vi "Main-Strech DNA-OneDirectionOnly_ver2_YCC.vi"(4 "Avg points":i32=120, 5 "Save Data?":bool, 6 "Who's Data":enum16{"YCC", "PYW", "LCH", "YYH"}(ring), 7 "Set LaserPower (mV)":dbl=-4500.0 format="%0.2f", 8 "File name add to the end \n(laser power-height)":string="FA-h300-1-1", 9 "Record scan rate  (um/s)":dbl=3.0 format="%.3f", 10 "range  (um)":dbl=2.9499999999999975 format="%.3f", 11 "T=X\nF=Y":bool=TRUE) -> (3 "Stage-QPD Graph":T4(graph))   [LabVIEW 2014]
uses:
  Main-Calibration/WLC fitting/SubVI/WLC-Fitting Cluster.ctl
  <vilib>/Analysis/baseanly.llb/Mean (DBL).vi
  <vilib>/Analysis/NI_AALBase.lvlib
panel:
  out "center":dbl
  out "avg. Step (nm)":dbl
  in  "WLC fitting?":bool
  in  "Force offset":dbl=800.0
  in  "Length offset":dbl=700.0
  in  "Filter type":T1(ring)=enum."F+S-window avg"
  in  "trap height(nm)":dbl=300.0
  out "Laser Lock?":bool
  in  "xDNA cut outside":dbl=3000.0
  in  "Fitting Cluster 2":T2={"cr (um)"=0.0, "yr (V)"=0.0, "trap height(nm)"=0.0, "bead radius(nm)"=520.0, "Length offset"=0.0, "Upper Force(pN)"=0.0, "cr shift (nm)"=0.0, "yr shift (mV)"=0.0, "LaserPower (mW)"=0.0, "conversion factor (V/um)"=0.0, "Stiffness (pN/nm)"=0.0154, "xDNA cut outside"=0.0, "Lower Force(pN)"=5.0, "c for zbd"=0.0}
  out "True rate?":bool
  in  "no fec":bool=TRUE
  in  "Avg. time delay (ms)":dbl=18.0
  in  "Use avg delay?":bool=TRUE
  out "delay time between F and U (ms)":dbl
  in  "no Record scan rate  (um/s)":dbl=2.0
  out "Fold QPD Signal (V) 2":dbl[](array[numeric])
  out "Fold Stage Position (um) 2":dbl[](array[numeric])
  out "Folded-Force":dbl[](array[numeric])
  out "Folded-xDNA":dbl[](array[numeric])
  out "Unfolded-Force":dbl[](array[numeric])
  out "Unfolded-xDNA":dbl[](array[numeric])
  out "Filtered QPD Array":dbl[][](array[numeric])
  out "Filtered Stage Array":dbl[][](array[numeric])
  out "Save to File Name Indicator":string
  out "Save to Path Indicator":path
  out "initial position offset after move":dbl[](array[numeric])
  out "Avg. to Hz":dbl
  out "Fold QPD Signal (V)":dbl[](array[numeric])
  out "Unfold QPD Signal (V)":dbl[](array[numeric])
  out "Fold Stage Position (um)":dbl[](array[numeric])
  out "Unfold Stage Position (um)":dbl[](array[numeric])
  in  "Tab Control":T3(tab)
  out "Stage-QPD Graph 3":T4(graph)
  out "Stage-QPD Graph 2":T4(graph)
  out "Unfolded Graph":cluster{dbl[], dbl[]}(graph)
  out "Folded Graph":cluster{dbl[], dbl[]}(graph)
  out "Unfolded+Folded Graph":T5(graph)
  out "Unfolded Fitting Graph":T6(graph)
  in  "initial parameters for eWLC (Lp,Lc,K)":dbl[](array[numeric])=[45.0, 1800.0, 1200.0]
  in  "initial parameters for marko (Lp,Lc)":dbl[](array[numeric])=[40.0, 1800.0]
  out "best fit parameters\n(Lp,Lc)":dbl[](array[numeric])
  out "best fit parameters\n(Lp,Lc,K)":dbl[](array[numeric])
  out "r^2":dbl
  out "r^2  2":dbl
  in  "eWLC?":bool
  out "Trace direction":bool[](array[boolean])=[FALSE, TRUE, TRUE, FALSE]
  out "Real initial position (um)":dbl format="%0.5f"
  in  "Toward first ?\nT=+, F=-":bool
  in  "Record Mode \npath(1,2)":bool[](array[boolean])=[TRUE, TRUE, FALSE, FALSE]
  in  "Sampling rate":dbl=32000.0 format="%0.2f"
  # "3.8 for full range"
  # "range=3.1um & 4 um/s\n-2000 m¢ä for activead"
  # "avg delay= 33ms\n20181223 ·s¬°18ms"
  # "3281-h300-sp40-RecA-ATPrS-6"
  # "3281-h300-m51 BRC4 2uM-Ca-ATP-1-8"
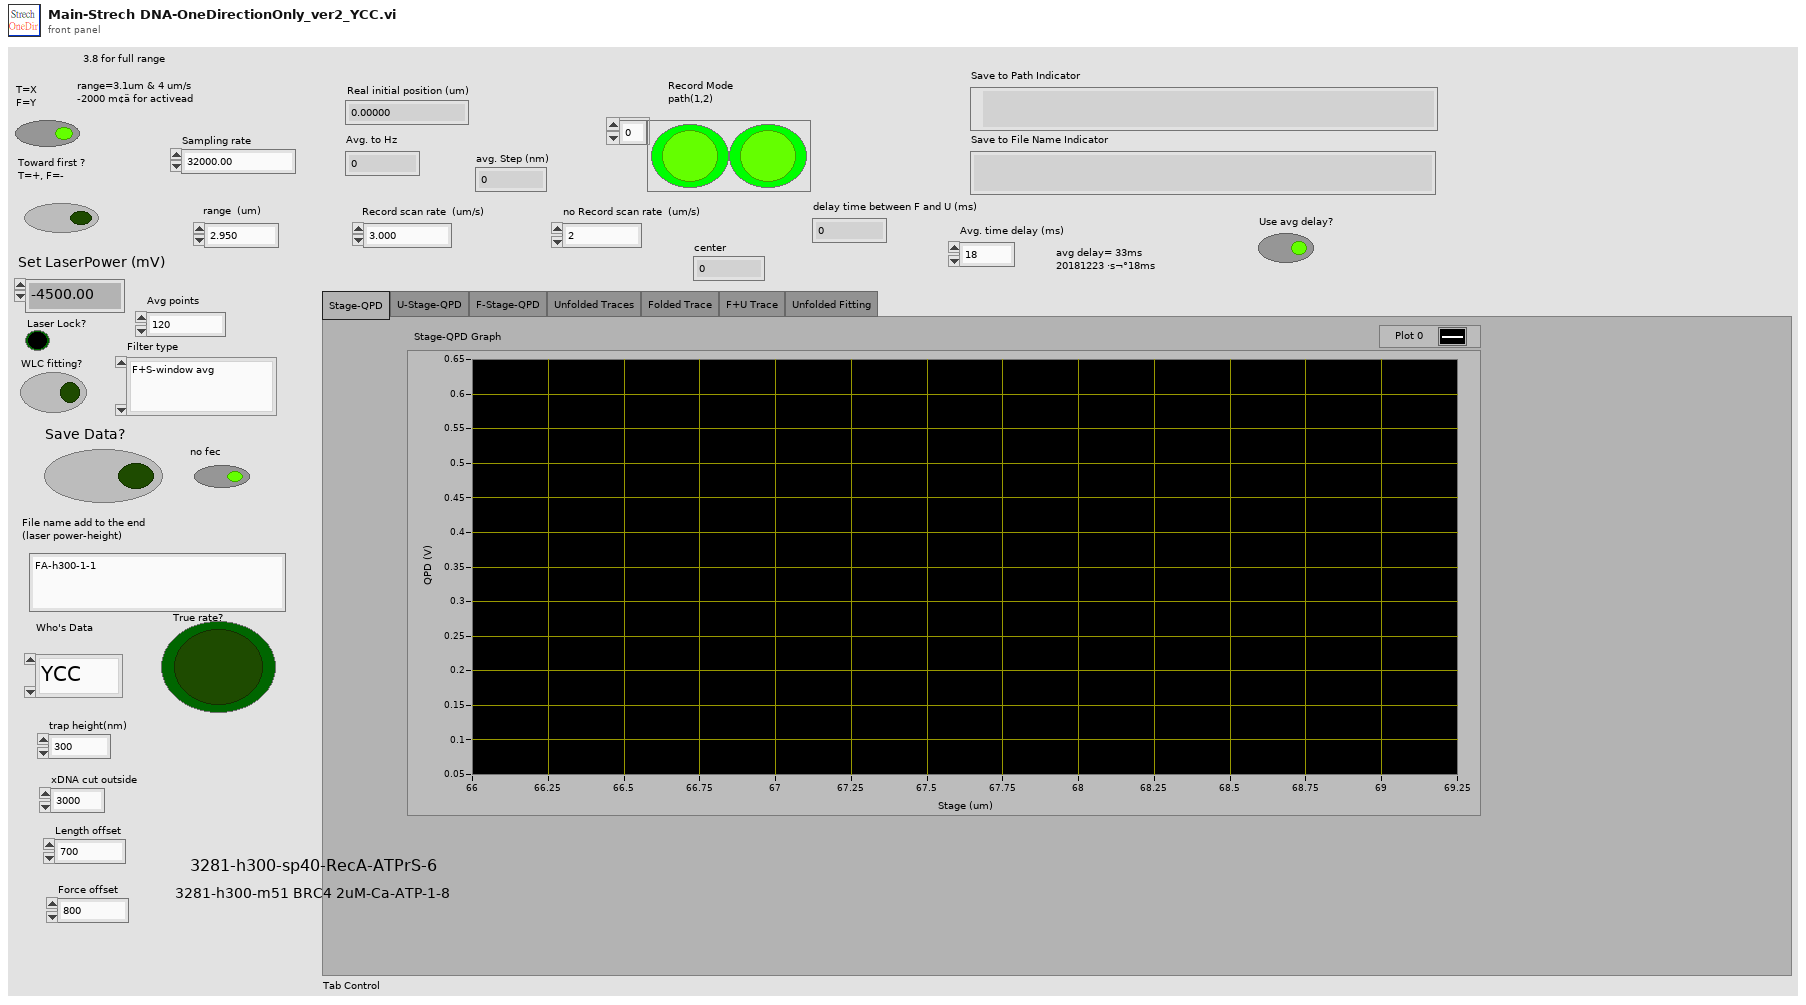
[diagram p1: front panel]
types:
  T1 = enum16{"Fixed-window avg", "Moving-window avg", "F+S-window avg", "S-G filter", "Fixed-window Median", "Moving-window Median "}
  T2 = typedef "WLC-Fitting Cluster.ctl" = cluster{"cr (um)":dbl, "yr (V)":dbl, "trap height(nm)":dbl, "bead radius(nm)":dbl, "Length offset":dbl, "Upper Force(pN)":dbl, "cr shift (nm)":dbl, "yr shift (mV)":dbl, "LaserPower (mW)":dbl, "conversion factor (V/um)":dbl, "Stiffness (pN/nm)":dbl, "xDNA cut outside":dbl, "Lower Force(pN)":dbl, "c for zbd":dbl}
  T3 = enum32{"Stage-QPD", "U-Stage-QPD", "F-Stage-QPD", "Unfolded Traces", "Folded Trace", "F+U Trace", "Unfolded Fitting"}
  T4 = cluster{"Fold Stage Position (um)":dbl[], "Fold QPD Signal (V)":dbl[]}
  T5 = cluster{"Filtered Stage Array":dbl[], "Filtered QPD Array":dbl[]}[]
  T6 = cluster{"best nonlinear fit for Extension (nm)":dbl[], "Force to fit":dbl[]}[]
  T7 = enum16{"Custom", "Centering", "1000 mV", "4500 mV"}
  T8 = cluster{"best nonlinear fit for Extension (nm)":dbl[], "Force to fit":dbl[]}
  T9 = cluster{"Unfolded-xDNA":dbl[], "Unfolded-Force":dbl[]}
  T10 = cluster{"Extension to fit":dbl[], "best nonlinear fit for Force (pN)":dbl[]}
  T11 = cluster{"Folded-xDNA":dbl[], "Folded-Force":dbl[]}
  T12 = cluster{"Folded-xDNA":dbl[], "Folded-Force":dbl[]}[]
  T13 = cluster{"Unfold Stage Position (um)":dbl[], "Unfold QPD Signal (V)":dbl[]}
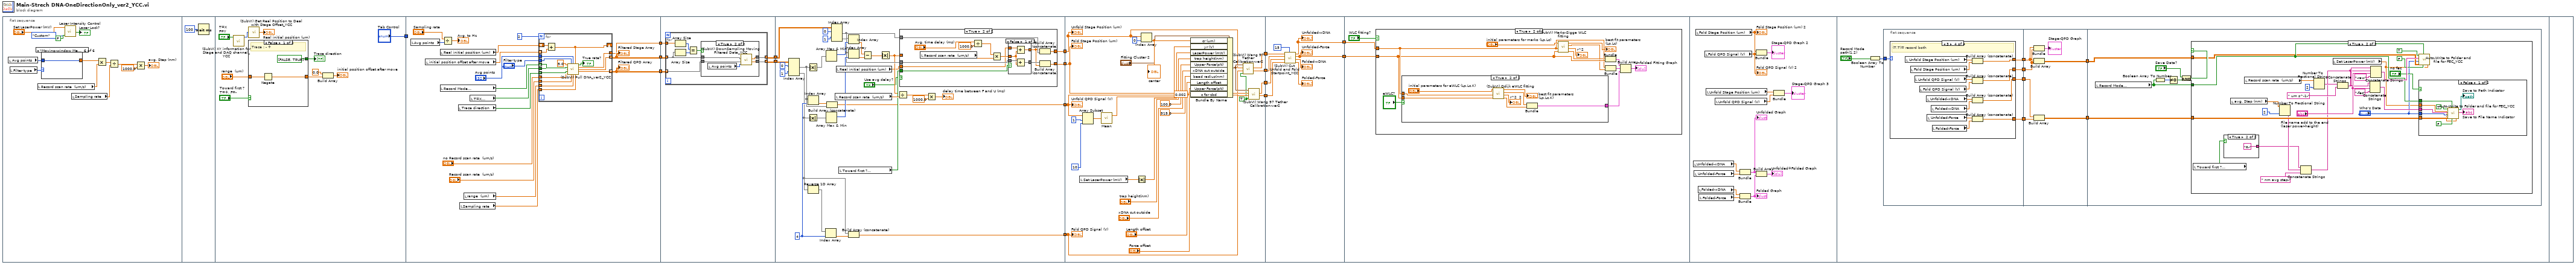
[diagram p0: block diagram]
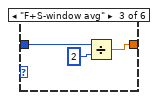
[diagram p4: hidden frame]
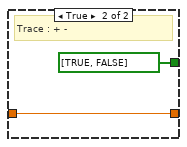
[diagram p7: hidden frame]
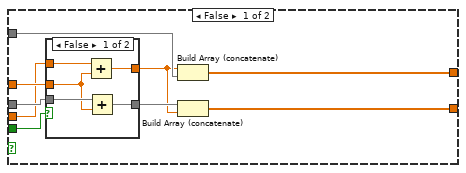
[diagram p9: hidden frame]
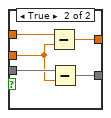
[diagram p10: hidden frame]
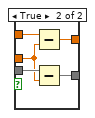
[diagram p11: hidden frame]
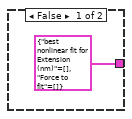
[diagram p13: hidden frame]
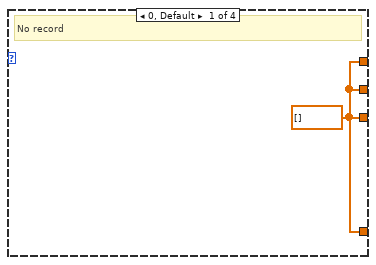
[diagram p14: hidden frame]
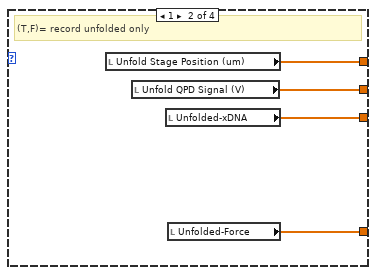
[diagram p15: hidden frame]
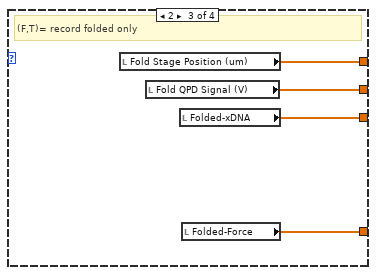
[diagram p16: hidden frame]
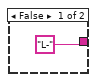
[diagram p18: hidden frame]
diagram:
  n1 = flat-sequence {
    tunnel: ["Tab Control"] -> w16
    tunnel: [w62] -> w5
    tunnel: [w61] -> w7
    tunnel: w16 -> [_]
    tunnel: [w54] -> w3
    tunnel: w7 -> [w92]
    tunnel: [w89] -> w6
    tunnel: w5 -> [w93]
    tunnel: [w90] -> w4
    tunnel: w3 -> [w91]
    tunnel: w6 -> [w136]
    tunnel: w4 -> [w139]
    tunnel: [w121] -> w11
    tunnel: [w116] -> w10
    tunnel: [w115] -> w9
    tunnel: [w118] -> w8
    tunnel: [w207] -> w15
    tunnel: [w206] -> w14
    tunnel: [w205] -> w13
    tunnel: [w204] -> w12
    tunnel: w11 -> [w203]
    tunnel: w10 -> [w192]
    tunnel: w9 -> [w202]
    tunnel: w8 -> [w193]
    tunnel: w15 -> [w218]
    tunnel: w14 -> [w217]
    tunnel: w13 -> [w216]
    tunnel: w12 -> [w214]
    tunnel: [w211] -> w2
    tunnel: [w210] -> w1
    tunnel: w2 -> [w221]
    tunnel: w1 -> [w220]
    frame #0 {
      n2 = local read "Avg points"() -> (w18:i32)
      n3 = local read "Filter type"() -> (w20:T1)
      n4 = local read "Record scan rate  (um/s)"() -> (w26:dbl)
      n5 = case shown="\"Moving-window Median \"" w20 {
        tunnel: [w30 w31 w32 w35 w36 w37] -> w19
        tunnel: w18 -> [w30 w31 w34 w35 w36 w37]
        frame "Fixed-window avg", Default {
        }
        frame "Moving-window avg" {
        }
        frame "F+S-window avg" {
          n6 = Divide(x=w34, y=2) -> (x/y=w32:dbl)
        }
        frame "S-G filter" {
        }
        frame "Fixed-window Median" {
        }
        frame "Moving-window Median " {
        }
      }
      n7 = call "Laser Intensity Control.vi"("Close?"=FALSE, "Enum"=T7."Custom", "Intensity Control, 0~-7000 (mV)"="Set LaserPower (mV)") -> ("Laser Lock?"=→"Laser Lock?":bool)  [unwired: 4 in]
      n8 = local read "Sampling rate"() -> (w24:dbl)
      n9 = Multiply(x=w19, y=w26) -> (x*y=w25:dbl)
      n10 = Divide(x=w25, y=w24) -> (x/y=w23:dbl)
      n11 = Multiply(x=w23, y=1000.0) -> (x*y=→"avg. Step (nm)":dbl)
    }
    frame #1 {
      n12 = Wait (ms)(milliseconds to wait=u32 100) -> ()  [unwired: 1 out]
    }
    frame #2 {
      n13 = call "(SubVI) XY information for Stage and DAQ channel_YCC.vi"("T=X\nF=Y"="T=X\nF=Y") -> ("Axis"=w46:i32)  [unwired: 3 in, 1 out]
      n14 = call "(SubVI) Get Real Position to Deal with Stage Offset_YCC.vi"("Axis"=w46) -> ("Real Current Commanded position (um)"=→"Real initial position (um)":dbl)  [unwired: 3 in, 1 out]
      n15 = case shown="False" "Toward first ?\nT=+, F=-" {
        tunnel: [bool[] [FALSE, TRUE] bool[] [TRUE, FALSE]] -> w44
        tunnel: "range  (um)" -> [w50 w52]
        tunnel: [w49 w52] -> w39
        frame False {
          # "Trace : - +"
          n16 = Negate(x=w50) -> (-x=w49:dbl)
        }
        frame True {
          # "Trace : + -"
        }
      }
      "Trace direction" <- w44
      n17 = Build Array(0.0, w39) -> (→"initial position offset after move":dbl[])
    }
    frame #3 {
      n18 = local read "Avg points"() -> (w66:i32)
      n19 = local read "initial position offset after move"() -> (w63:dbl[])
      n20 = local read "Real initial position (um)"() -> (w57:dbl)
      n21 = local read "Record Mode \npath(1,2)"() -> (w68:bool[])
      n22 = Divide(x="Sampling rate", y=w66) -> (x/y=→"Avg. to Hz":dbl)
      n23 = local read "Trace direction"() -> (w69:bool[])
      n24 = local read "Sampling rate"() -> (w58:dbl)
      n25 = local read "range  (um)"() -> (w64:dbl)
      n26 = local read "T=X\nF=Y"() -> (w70:bool)
      n27 = for {
        N: 2 -> [_]
        tunnel: "Avg points" -> [w88]
        tunnel: w68 -> [w87] mode=indexing
        tunnel: w70 -> [w86]
        tunnel: w69 -> [w79] mode=indexing
        tunnel: w58 -> [w85]
        tunnel: "Record scan rate  (um/s)" -> [w84]
        tunnel: w64 -> [w83]
        tunnel: [w73] -> w62 mode=indexing
        tunnel: [w74] -> w61 mode=indexing
        shift-right: [w80] -> _
        shift-left: w57 -> [w81]
        tunnel: w63 -> [w82] mode=indexing
        tunnel: "no Record scan rate  (um/s)" -> [w78]
        tunnel: "Filter type" -> [w75]
        tunnel: [w72] -> w54
        n28 = Add(x=w81, y=w82) -> (x+y=w80:dbl)
        n29 = call "(SubVI) Pull DNA_ver2_YCC.vi"("waiting time per point (ms)\nrange from 5ms to 0.167 ms"=5.0 ("waiting time per point (ms)\nrange from 5ms to 0.167 ms"), "Filter type"=w75, "Avg points"=w88, "Real initial position (um)"=w80, "Record?"=w87, "T=X\nF=Y"=w86, "Toward  ?\nT=+, F=-"=w79, "no Record scan rate  (um/s)"=w78, "Record scan rate  (um/s)"=w84, "range  (um)"=w83, "Sampling rate"=w85) -> ("True rate?"=→"True rate?":bool, "Raw Stage Array"=w72:dbl[], "Filtered Stage Array"=w73:dbl[], "Filtered QPD Array"=w74:dbl[])  [unwired: 1 in]
      }
      "Filtered Stage Array" <- w62
      "Filtered QPD Array" <- w61
    }
    frame #4 {
      n30 = for {
        tunnel: w93 -> [w96] mode=indexing
        tunnel: w92 -> [w98] mode=indexing
        tunnel: w91 -> [w97]
        tunnel: [w95] -> w90 mode=indexing
        tunnel: [w94] -> w89 mode=indexing
        n31 = Array Size(array=w97) -> (size(s)=w99:i32)
        n32 = Array Size(array=w96) -> (size(s)=w100:i32)
        n33 = Equal?(x=w99, y=w100) -> (x = y?=w101:bool)
        n34 = case shown="True" w101 {
          tunnel: w96 -> [w103 w107]
          tunnel: w98 -> [w102 w106]
          tunnel: [w102 w105] -> w94
          tunnel: [w103 w104] -> w95
          frame False {
          }
          frame True {
            n35 = local read "Avg points"() -> (w108:i32)
            n36 = call "(SubVI) DownSampling Moving Filtered Data_YCC.vi"("data# reduce factor"=w108, "Moving Filtered QPD data"=w106, "Moving Filtered Stage data"=w107) -> ("DownSampling QPD"=w105:dbl[], "DownSampling Stage"=w104:dbl[])  [unwired: 3 in]
          }
        }
      }
    }
    frame #5 {
      w113 = 4 ("index")
      n37 = Index Array(array=w136, index (row) #1=0 ("index (row)"), index (row) #2=1 ("index (row)")) -> (element #1=w114:dbl[], element #2=w110:dbl[])  [unwired: 2 in]
      n38 = Absolute Value(x=w114) -> (abs(x)=w135:dbl[])
      n39 = Absolute Value(x=w110) -> (abs(x)=w134:dbl[])
      n40 = Index Array(array=w114, index=w113) -> (element=w112:dbl)
      n41 = Reverse 1D Array(array=w110) -> (reversed array=w109:dbl[])
      n42 = Index Array(array=w109, index=w113) -> (element=w111:dbl)
      n43 = Array Max & Min(array=w135) -> (max index (indices)=w131:i32)  [unwired: 3 out]
      n44 = Array Max & Min(array=w134) -> (max index (indices)=w130:i32)  [unwired: 3 out]
      n45 = Build Array (concatenate)(w112, w114) -> (w116:dbl[])
      n46 = Index Array(array=w139, index (row) #1=0 ("index (row)"), index (row) #2=1 ("index (row)")) -> (element #1=w119:dbl[], element #2=w123:dbl[])  [unwired: 2 in]
      n47 = local read "Record scan rate  (um/s)"() -> (w125:dbl)
      n48 = local read "Real initial position (um)"() -> (w117:dbl)
      n49 = local read "Toward first ?\nT=+, F=-"() -> (w124:bool)
      n50 = Index Array(array=w119, index=w131) -> (element=w133:dbl)
      n51 = Index Array(array=w123, index=w130) -> (element=w132:dbl)
      n52 = Build Array (concatenate)(w110, w111) -> (w115:dbl[])
      n53 = Subtract(x=w133, y=w132) -> (x-y=w126:dbl)
      n54 = Absolute Value(x=w126) -> (abs(x)=w122:dbl)
      n55 = Divide(x=w122, y=w125) -> (x/y=w129:dbl)
      n56 = case shown="True" "Use avg delay?" {
        tunnel: w124 -> [w150 w171]
        tunnel: w123 -> [w149 w172]
        tunnel: w122 -> [w148 _]
        tunnel: [w143 w162] -> w121
        tunnel: w119 -> [w147 w166]
        tunnel: [w146 w165] -> w118
        tunnel: w117 -> [w142 w161]
        frame False {
          n57 = case shown="False" w150 {
            tunnel: w149 -> [w155 w160]
            tunnel: w148 -> [w152 w157]
            tunnel: [w154 w159] -> w145
            tunnel: w142 -> [w153 w158]
            tunnel: [w151 w156] -> w144
            frame False {
              n58 = Add(x=w153, y=w152) -> (x+y=w151:dbl)
              n59 = Add(x=w155, y=w152) -> (x+y=w154:dbl[])
            }
            frame True {
              n60 = Subtract(x=w158, y=w157) -> (x-y=w156:dbl)
              n61 = Subtract(x=w160, y=w157) -> (x-y=w159:dbl[])
            }
          }
          n62 = Build Array (concatenate)(w144, w147) -> (w146:dbl[])
          n63 = Build Array (concatenate)(w145, w144) -> (w143:dbl[])
        }
        frame True {
          n64 = local read "Record scan rate  (um/s)"() -> (w173:dbl)
          n65 = Divide(x="Avg. time delay (ms)", y=1000.0) -> (x/y=w168:dbl)
          n66 = Multiply(x=w168, y=w173) -> (x*y=w170:dbl)
          n67 = case shown="False" w171 {
            tunnel: w172 -> [w178 w183]
            tunnel: w170 -> [w175 w180]
            tunnel: [w177 w182] -> w164
            tunnel: w161 -> [w176 w181]
            tunnel: [w174 w179] -> w163
            frame False {
              n68 = Add(x=w176, y=w175) -> (x+y=w174:dbl)
              n69 = Add(x=w178, y=w175) -> (x+y=w177:dbl[])
            }
            frame True {
              n70 = Subtract(x=w181, y=w180) -> (x-y=w179:dbl)
              n71 = Subtract(x=w183, y=w180) -> (x-y=w182:dbl[])
            }
          }
          n72 = Build Array (concatenate)(w163, w166) -> (w165:dbl[])
          n73 = Build Array (concatenate)(w164, w163) -> (w162:dbl[])
        }
      }
      n74 = Multiply(x=w129, y=1000.0) -> (x*y=→"delay time between F and U (ms)":dbl)
    }
    frame #6 {
      w185 = TRUE ("X=T\nY=F")
      n75 = local read "Set LaserPower (mV)"() -> (w197:dbl)
      n76 = Array Subset(array=w192, index=1, length=10) -> (w189:dbl[])
      n77 = call-poly <vilib>:"Mean.vi"("X"=w189) -> ("mean"=w188:dbl)  [unwired: 1 out]
      n78 = Absolute Value(x=w197) -> (abs(x)=w196:dbl)
      n79 = Index Array(array=w193, index=0) -> (element=w208:dbl)
      "center" <- w208
      n80 = Bundle By Name(cluster="Fitting Cluster 2", "cr (um)"=w208, "yr (V)"=w188, "LaserPower (mW)"=w196, "trap height(nm)"="trap height(nm)", "Upper Force(pN)"=100.0 ("Force offset"), "xDNA cut outside"="xDNA cut outside", "bead radius(nm)"=515.0, "Length offset"="Length offset", "Upper Force(pN)"="Force offset", "c for zbd"=0.002) -> (w200:T2)
      n81 = call "(SubVI) Wang 97 Tether Calibration-ver2.vi"("X=T\nY=F"=w185, "QPD signal"=w192, "Stage Position"=w193, "Fitting Cluster"=w200) -> ("Force"=w206:dbl[], "xDNA"=w207:dbl[])  [unwired: 1 in, 1 out]
      n82 = call "(SubVI) Wang 97 Tether Calibration-ver2.vi"("X=T\nY=F"=w185, "QPD signal"=w202, "Stage Position"=w203, "Fitting Cluster"=w200) -> ("Force"=w204:dbl[], "xDNA"=w205:dbl[])  [unwired: 1 in, 1 out]
      "Unfold Stage Position (um)" <- w193
      "Fold Stage Position (um)" <- w203
      "Unfold QPD Signal (V)" <- w192
      "Fold QPD Signal (V)" <- w202
    }
    frame #7 {
      n83 = call "(SubVI) Cut Unfold and Fold Startpoint_YCC.vi"("number to cut"=15, "Folded-Force in"=w214, "Folded-xDNA in"=w216, "Unfolded-Force"=w217, "Unfolded-xDNA"=w218) -> ("Folded-Force"=→"Folded-Force":dbl[], "Folded-xDNA"=→"Folded-xDNA":dbl[], "Unfolded-Force"=w210:dbl[], "Unfolded-xDNA"=w211:dbl[])  [unwired: 3 in]
      "Unfolded-Force" <- w210
      "Unfolded-xDNA" <- w211
    }
    frame #8 {
      n84 = case shown="True" "WLC fitting?" {
        tunnel: w221 -> [_ w230]
        tunnel: w220 -> [_ w229]
        frame False {
        }
        frame True {
          n85 = case shown="True" "eWLC?" {
            tunnel: w230 -> [_ w239]
            tunnel: w229 -> [_ w238]
            tunnel: [T8 {"best nonlinear fit for Extension (nm)"=[], "Force to fit"=[]} w235] -> w224
            frame False {
            }
            frame True {
              n86 = call "(SubVI) Odijk eWLC fitting.vi"("Force (pN)"=w238, "Extension (nm)"=w239, "initial parameters for eWLC (Lp,Lc,K=1200)"="initial parameters for eWLC (Lp,Lc,K)") -> ("Force to fit"=w236:dbl[], "r^2"=→"r^2  2":dbl, "best nonlinear fit for Extension (nm)"=w237:dbl[], "best fit parameters\n(Lp,Lc,K=1200)"=→"best fit parameters\n(Lp,Lc,K)":dbl[])  [unwired: 1 in]
              n87 = Bundle("best nonlinear fit for Extension (nm)"=w237, "Force to fit"=w236) -> (w235:T8)  [unwired: 1 in]
            }
          }
          n88 = call "(SubVI) Marko-Sigga WLC fitting.vi"("Force (pN)"=w229, "Extension (nm)"=w230, "initial parameters for marko"="initial parameters for marko (Lp,Lc)") -> ("Extension to fit"=w228:dbl[], "r^2"=→"r^2":dbl, "best nonlinear fit for Force (pN)"=w227:dbl[], "best fit parameters\n(Lp,Lc)"=→"best fit parameters\n(Lp,Lc)":dbl[])  [unwired: 1 in]
          n89 = Bundle("Unfolded-xDNA"=w230, "Unfolded-Force"=w229) -> (w226:T9)  [unwired: 1 in]
          n90 = Bundle("Extension to fit"=w228, "best nonlinear fit for Force (pN)"=w227) -> (w225:T10)  [unwired: 1 in]
          n91 = Build Array(w226, w225, w224) -> (→"Unfolded Fitting Graph":T6)
        }
      }
    }
    frame #9 {
      n92 = local read "Unfolded-xDNA"() -> (w255:dbl[])
      n93 = local read "Unfolded-Force"() -> (w254:dbl[])
      n94 = local read "Fold Stage Position (um)"() -> (w247:dbl[])
      "Fold Stage Position (um) 2" <- w247
      n95 = local read "Folded-xDNA"() -> (w252:dbl[])
      n96 = local read "Folded-Force"() -> (w251:dbl[])
      n97 = local read "Fold QPD Signal (V)"() -> (w246:dbl[])
      "Fold QPD Signal (V) 2" <- w246
      n98 = local read "Unfold Stage Position (um)"() -> (w245:dbl[])
      n99 = local read "Unfold QPD Signal (V)"() -> (w244:dbl[])
      n100 = Bundle("Unfolded-xDNA"=w255, "Unfolded-Force"=w254) -> (w253:T9)  [unwired: 1 in]
      "Unfolded Graph" <- w253
      n101 = Bundle("Folded-xDNA"=w252, "Folded-Force"=w251) -> (w249:T11)  [unwired: 1 in]
      "Folded Graph" <- w249
      n102 = Bundle("Fold Stage Position (um)"=w247, "Fold QPD Signal (V)"=w246) -> (→"Stage-QPD Graph 2":T4)  [unwired: 1 in]
      n103 = Build Array(w253, w249) -> (→"Unfolded+Folded Graph":T12)
      n104 = Bundle("Unfold Stage Position (um)"=w245, "Unfold QPD Signal (V)"=w244) -> (→"Stage-QPD Graph 3":T13)  [unwired: 1 in]
    }
    frame #10 {
      n105 = Boolean Array To Number(Boolean array="Record Mode \npath(1,2)") -> (number=w262:u32)
      n106 = flat-sequence {
        tunnel: w262 -> [w266]
        tunnel: [w268] -> w261
        tunnel: [w267] -> w260
        tunnel: [w265] -> w258
        tunnel: [w264] -> w257
        tunnel: w261 -> [w292]
        tunnel: w260 -> [w291]
        tunnel: [w296] -> w259
        tunnel: w258 -> [w295]
        tunnel: w257 -> [w294]
        tunnel: [w293] -> w256
        tunnel: w259 -> [w300]
        tunnel: w256 -> [w297]
        frame #0 {
          n107 = case shown="3" w266 {
            tunnel: [w269 w273 w277 w285] -> w268
            tunnel: [w269 w272 w276 w284] -> w267
            tunnel: [w269 w271 w275 w279] -> w265
            tunnel: [w269 w270 w274 w278] -> w264
            frame 0, Default {
              w269 = dbl[] [] ("Fold Stage Position (um)")
              # "No record"
            }
            frame 1 {
              # "(T,F)= record unfolded only"
              n108 = local read "Unfold Stage Position (um)"() -> (w273:dbl[])
              n109 = local read "Unfold QPD Signal (V)"() -> (w272:dbl[])
              n110 = local read "Unfolded-xDNA"() -> (w271:dbl[])
              n111 = local read "Unfolded-Force"() -> (w270:dbl[])
            }
            frame 2 {
              # "(F,T)= record folded only"
              n112 = local read "Fold Stage Position (um)"() -> (w277:dbl[])
              n113 = local read "Fold QPD Signal (V)"() -> (w276:dbl[])
              n114 = local read "Folded-xDNA"() -> (w275:dbl[])
              n115 = local read "Folded-Force"() -> (w274:dbl[])
            }
            frame 3 {
              # "(T,T)= record both"
              n116 = local read "Unfold Stage Position (um)"() -> (w289:dbl[])
              n117 = local read "Fold Stage Position (um)"() -> (w288:dbl[])
              n118 = local read "Unfold QPD Signal (V)"() -> (w287:dbl[])
              n119 = local read "Fold QPD Signal (V)"() -> (w286:dbl[])
              n120 = local read "Unfolded-xDNA"() -> (w283:dbl[])
              n121 = local read "Unfolded-Force"() -> (w281:dbl[])
              n122 = local read "Folded-xDNA"() -> (w282:dbl[])
              n123 = local read "Folded-Force"() -> (w280:dbl[])
              n124 = Build Array (concatenate)(w289, w288) -> (w285:dbl[])
              n125 = Build Array (concatenate)(w287, w286) -> (w284:dbl[])
              n126 = Build Array (concatenate)(w283, w282) -> (w279:dbl[])
              n127 = Build Array (concatenate)(w281, w280) -> (w278:dbl[])
            }
          }
        }
        frame #1 {
          n128 = Bundle("Fold Stage Position (um)"=w292, "Fold QPD Signal (V)"=w291) -> (→"Stage-QPD Graph":T4)  [unwired: 1 in]
          n129 = Build Array(w292, w291) -> (w296:dbl[][])
          n130 = Build Array(w295, w294) -> (w293:dbl[][])
        }
        frame #2 {
          n131 = local read "Record Mode \npath(1,2)"() -> (w298:bool[])
          n132 = Boolean Array To Number(Boolean array=w298) -> (number=w299:u32)
          n133 = Not Equal To 0?(x=w299) -> (x != 0?=w302:bool)
          n134 = And(x="Save Data?", y=w302) -> (x .and. y?=w301:bool)
          n135 = case shown="True" w301 {
            tunnel: w300 -> [_ w320]
            tunnel: w298 -> [_ w322]
            tunnel: w297 -> [_ w321]
            frame False {
            }
            frame True {
              n136 = local read "Toward first ?\nT=+, F=-"() -> (w305:bool)
              n137 = case shown="True" w305 {
                tunnel: ["L-" "R-"] -> w304
                frame False {
                }
                frame True {
                }
              }
              n138 = local read "avg. Step (nm)"() -> (w310:dbl)
              n139 = local read "Record scan rate  (um/s)"() -> (w316:dbl)
              n140 = Number To Fractional String(number=w310, precision (6)=i16 2) -> (F-format string=w308:string)  [unwired: 2 in]
              n141 = Concatenate Strings(w304, w308, " nm avg step-") -> (w306:string)
              n142 = Number To Fractional String(number=w316, precision (6)=i16 2) -> (F-format string=w317:string)  [unwired: 2 in]
              n143 = local read "Set LaserPower (mV)"() -> (w312:dbl)
              n144 = Concatenate Strings(w317, " um s^-1-") -> (w311:string)
              n145 = Concatenate Strings(w311, w306, "File name add to the end \n(laser power-height)", "-fec" ("string")) -> (w326:string)
              n146 = Concatenate Strings(w311, w306, "File name add to the end \n(laser power-height)", "-raw" ("string")) -> (w323:string)
              n147 = call "Auto-Write to Folder and file for FEC_YCC.vi"("Current PD (mV)"=w312, "Centering data?"=FALSE, "Record Mode \npath(1,2)"=w322, "data to be saved"=w320, "Who's Data"="Who's Data", "File name add to the end \n(height)"=w323, "Save?"=TRUE) -> ()  [unwired: 1 in, 2 out]
              n148 = case shown="False" "no fec" {
                tunnel: w326 -> [w336 _]
                tunnel: w322 -> [w335 _]
                tunnel: w321 -> [w334 _]
                tunnel: "Who's Data" -> [w332 _]
                tunnel: w312 -> [w331 _]
                frame False {
                  n149 = call "Auto-Write to Folder and file for FEC_YCC.vi"("Current PD (mV)"=w331, "Centering data?"=FALSE, "Record Mode \npath(1,2)"=w335, "data to be saved"=w334, "Who's Data"=w332, "File name add to the end \n(height)"=w336, "Save?"=TRUE) -> ("Save to File Name"=→"Save to File Name Indicator":string, "Save to Path"=→"Save to Path Indicator":path)  [unwired: 1 in]
                }
                frame True {
                }
              }
            }
          }
        }
      }
    }
    frame #11 {
    }
  }
